vi "main(Test DQMH modules).vi"() -> ()   [LabVIEW 2018, in "Application.lvlib"] (continued)
              n2421 = call "App enquece.vi"("Priority Enquece"=TRUE, "command data"=w5478, "command"=w5479, "queue in"=w5481) -> ("error out"=w5482:errorcluster)  [unwired: 6 in, 1 out]
            }
          }
          frame True {
          }
        }
        n2422 = Merge Errors(w5454, w5456) -> (w5455:errorcluster)
      }
      frame "Test DRV 47" {
        w5488 = 47  # DUT index(0-59)
        n2423 = disable-structure shown="LOGGING==TRUE" {
          disable-tunnel: w5490 -> [w5525 _]
          frame condition #0 (active) {
            n2424 = Empty String/Path?(string/path=w5525) -> (empty?=w5528:bool)
            n2425 = Select(t="Quece timeout", s=w5528, f=w5525) -> (s? t:f=w5524:string)
            n2426 = call "string log (SubVI).vi"("Enum"=enum16{"Init", "Log", "Read"}."Log", "state Name"=w5524) -> ()  [unwired: 8 in, 2 out]
          }
          frame condition #1 {
          }
        }
        n2427 = call "progress string(SubVI).vi"("String 3"=w5490, "String in"=w5491) -> ("String out"=w5492:string)  [unwired: 9 in]
        n2428 = call "FGV Driver Data.vi"("DUT index(1-60)"=w5488) -> ("DUT SC"=w5489:bool)  [unwired: 7 in, 3 out]
        n2429 = case shown="False" w5489 {
          tunnel: [w5517 _] -> w5497
          tunnel: w5494 -> [w5516 _]
          frame False {
            w5504 = T11 {"command"="", "command data"=variant} ("element")
            w5503 = "MEAS.mux6_1"
            n2430 = To Variant(anything=T4."mux6-1_channel0" ("mux6_1(3wires)_encode")) -> (Variant=w5502:variant)
            n2431 = To Variant(anything=T4."mux6_1_channel5_3" ("mux6_1(3wires)_encode")) -> (Variant=w5514:variant)
            n2432 = To Variant(anything=T4."mux6_1_channel5_2" ("mux6_1(3wires)_encode")) -> (Variant=w5512:variant)
            n2433 = Bundle By Name(cluster=w5504, "command"=w5503, "command data"=w5512) -> (w5511:T11)
            n2434 = Bundle By Name(cluster=w5504, "command"=w5503, "command data"=w5514) -> (w5510:T11)
            n2435 = Bundle By Name(cluster=w5504, "command"=w5503, "command data"=w5502) -> ()  [unwired: 1 out]
            n2436 = Bundle By Name(cluster=w5504, "command"="MEAS.DMM dual read") -> (w5508:T11)
            n2437 = Build Array(w5511, w5510, w5508) -> (w5506:T11[])
            n2438 = Reverse 1D Array(array=w5506) -> (reversed array=w5507:T11[])
            n2439 = for {
              tunnel: [w5523] -> w5517 mode=indexing
              tunnel: w5516 -> [w5522]
              tunnel: w5507 -> [w5521] mode=indexing
              n2440 = Unbundle By Name(w5521) -> ("command"=w5520:string, "command data"=w5519:variant)
              n2441 = call "App enquece.vi"("Priority Enquece"=TRUE, "command data"=w5519, "command"=w5520, "queue in"=w5522) -> ("error out"=w5523:errorcluster)  [unwired: 6 in, 1 out]
            }
          }
          frame True {
          }
        }
        n2442 = Merge Errors(w5495, w5497) -> (w5496:errorcluster)
      }
      frame "Test DRV 48" {
        w5530 = 48  # DUT index(0-59)
        n2443 = disable-structure shown="LOGGING==TRUE" {
          disable-tunnel: w5531 -> [w5566 _]
          frame condition #0 (active) {
            n2444 = Empty String/Path?(string/path=w5566) -> (empty?=w5569:bool)
            n2445 = Select(t="Quece timeout", s=w5569, f=w5566) -> (s? t:f=w5565:string)
            n2446 = call "string log (SubVI).vi"("Enum"=enum16{"Init", "Log", "Read"}."Log", "state Name"=w5565) -> ()  [unwired: 8 in, 2 out]
          }
          frame condition #1 {
          }
        }
        n2447 = call "progress string(SubVI).vi"("String 3"=w5531, "String in"=w5532) -> ("String out"=w5533:string)  [unwired: 9 in]
        n2448 = call "FGV Driver Data.vi"("DUT index(1-60)"=w5530) -> ("DUT SC"=w5529:bool)  [unwired: 7 in, 3 out]
        n2449 = case shown="False" w5529 {
          tunnel: [w5558 _] -> w5538
          tunnel: w5535 -> [w5557 _]
          frame False {
            w5545 = T11 {"command"="", "command data"=variant} ("element")
            w5544 = "MEAS.mux6_1"
            n2450 = To Variant(anything=T4."mux6-1_channel0" ("mux6_1(3wires)_encode")) -> (Variant=w5543:variant)
            n2451 = To Variant(anything=T4."mux6_1_channel6_3" ("mux6_1(3wires)_encode")) -> (Variant=w5555:variant)
            n2452 = To Variant(anything=T4."mux6_1_channel6_2" ("mux6_1(3wires)_encode")) -> (Variant=w5553:variant)
            n2453 = Bundle By Name(cluster=w5545, "command"=w5544, "command data"=w5553) -> (w5552:T11)
            n2454 = Bundle By Name(cluster=w5545, "command"=w5544, "command data"=w5555) -> (w5551:T11)
            n2455 = Bundle By Name(cluster=w5545, "command"=w5544, "command data"=w5543) -> ()  [unwired: 1 out]
            n2456 = Bundle By Name(cluster=w5545, "command"="MEAS.DMM dual read") -> (w5549:T11)
            n2457 = Build Array(w5552, w5551, w5549) -> (w5547:T11[])
            n2458 = Reverse 1D Array(array=w5547) -> (reversed array=w5548:T11[])
            n2459 = for {
              tunnel: [w5564] -> w5558 mode=indexing
              tunnel: w5557 -> [w5563]
              tunnel: w5548 -> [w5562] mode=indexing
              n2460 = Unbundle By Name(w5562) -> ("command"=w5561:string, "command data"=w5560:variant)
              n2461 = call "App enquece.vi"("Priority Enquece"=TRUE, "command data"=w5560, "command"=w5561, "queue in"=w5563) -> ("error out"=w5564:errorcluster)  [unwired: 6 in, 1 out]
            }
          }
          frame True {
          }
        }
        n2462 = Merge Errors(w5536, w5538) -> (w5537:errorcluster)
      }
      frame "Test DRV 49" {
        w5570 = 49  # DUT index(0-59)
        n2463 = disable-structure shown="LOGGING==TRUE" {
          disable-tunnel: w5572 -> [w5607 _]
          frame condition #0 (active) {
            n2464 = Empty String/Path?(string/path=w5607) -> (empty?=w5610:bool)
            n2465 = Select(t="Quece timeout", s=w5610, f=w5607) -> (s? t:f=w5606:string)
            n2466 = call "string log (SubVI).vi"("Enum"=enum16{"Init", "Log", "Read"}."Log", "state Name"=w5606) -> ()  [unwired: 8 in, 2 out]
          }
          frame condition #1 {
          }
        }
        n2467 = call "progress string(SubVI).vi"("String 3"=w5572, "String in"=w5573) -> ("String out"=w5574:string)  [unwired: 9 in]
        n2468 = call "FGV Driver Data.vi"("DUT index(1-60)"=w5570) -> ("DUT SC"=w5571:bool)  [unwired: 7 in, 3 out]
        n2469 = case shown="False" w5571 {
          tunnel: [w5599 _] -> w5579
          tunnel: w5576 -> [w5598 _]
          frame False {
            w5586 = T11 {"command"="", "command data"=variant} ("element")
            w5585 = "MEAS.mux6_1"
            n2470 = To Variant(anything=T4."mux6-1_channel0" ("mux6_1(3wires)_encode")) -> (Variant=w5584:variant)
            n2471 = To Variant(anything=T4."mux6_1_channel1_3" ("mux6_1(3wires)_encode")) -> (Variant=w5596:variant)
            n2472 = To Variant(anything=T4."mux6-1_channel1_2" ("mux6_1(3wires)_encode")) -> (Variant=w5594:variant)
            n2473 = Bundle By Name(cluster=w5586, "command"=w5585, "command data"=w5594) -> (w5593:T11)
            n2474 = Bundle By Name(cluster=w5586, "command"=w5585, "command data"=w5596) -> (w5592:T11)
            n2475 = Bundle By Name(cluster=w5586, "command"=w5585, "command data"=w5584) -> ()  [unwired: 1 out]
            n2476 = Bundle By Name(cluster=w5586, "command"="MEAS.DMM dual read") -> (w5590:T11)
            n2477 = Build Array(w5593, w5592, w5590) -> (w5588:T11[])
            n2478 = Reverse 1D Array(array=w5588) -> (reversed array=w5589:T11[])
            n2479 = for {
              tunnel: [w5605] -> w5599 mode=indexing
              tunnel: w5598 -> [w5604]
              tunnel: w5589 -> [w5603] mode=indexing
              n2480 = Unbundle By Name(w5603) -> ("command"=w5602:string, "command data"=w5601:variant)
              n2481 = call "App enquece.vi"("Priority Enquece"=TRUE, "command data"=w5601, "command"=w5602, "queue in"=w5604) -> ("error out"=w5605:errorcluster)  [unwired: 6 in, 1 out]
            }
          }
          frame True {
          }
        }
        n2482 = Merge Errors(w5577, w5579) -> (w5578:errorcluster)
      }
      frame "Test DRV 50" {
        w5611 = 50  # DUT index(0-59)
        n2483 = disable-structure shown="LOGGING==TRUE" {
          disable-tunnel: w5613 -> [w5648 _]
          frame condition #0 (active) {
            n2484 = Empty String/Path?(string/path=w5648) -> (empty?=w5651:bool)
            n2485 = Select(t="Quece timeout", s=w5651, f=w5648) -> (s? t:f=w5647:string)
            n2486 = call "string log (SubVI).vi"("Enum"=enum16{"Init", "Log", "Read"}."Log", "state Name"=w5647) -> ()  [unwired: 8 in, 2 out]
          }
          frame condition #1 {
          }
        }
        n2487 = call "progress string(SubVI).vi"("String 3"=w5613, "String in"=w5614) -> ("String out"=w5615:string)  [unwired: 9 in]
        n2488 = call "FGV Driver Data.vi"("DUT index(1-60)"=w5611) -> ("DUT SC"=w5612:bool)  [unwired: 7 in, 3 out]
        n2489 = case shown="False" w5612 {
          tunnel: [w5640 _] -> w5620
          tunnel: w5617 -> [w5639 _]
          frame False {
            w5627 = T11 {"command"="", "command data"=variant} ("element")
            w5626 = "MEAS.mux6_1"
            n2490 = To Variant(anything=T4."mux6-1_channel0" ("mux6_1(3wires)_encode")) -> (Variant=w5625:variant)
            n2491 = To Variant(anything=T4."mux6_1_channel2_3" ("mux6_1(3wires)_encode")) -> (Variant=w5637:variant)
            n2492 = To Variant(anything=T4."mux6_1_channel2_2" ("mux6_1(3wires)_encode")) -> (Variant=w5635:variant)
            n2493 = Bundle By Name(cluster=w5627, "command"=w5626, "command data"=w5635) -> (w5634:T11)
            n2494 = Bundle By Name(cluster=w5627, "command"=w5626, "command data"=w5637) -> (w5633:T11)
            n2495 = Bundle By Name(cluster=w5627, "command"=w5626, "command data"=w5625) -> ()  [unwired: 1 out]
            n2496 = Bundle By Name(cluster=w5627, "command"="MEAS.DMM dual read") -> (w5631:T11)
            n2497 = Build Array(w5634, w5633, w5631) -> (w5629:T11[])
            n2498 = Reverse 1D Array(array=w5629) -> (reversed array=w5630:T11[])
            n2499 = for {
              tunnel: [w5646] -> w5640 mode=indexing
              tunnel: w5639 -> [w5645]
              tunnel: w5630 -> [w5644] mode=indexing
              n2500 = Unbundle By Name(w5644) -> ("command"=w5643:string, "command data"=w5642:variant)
              n2501 = call "App enquece.vi"("Priority Enquece"=TRUE, "command data"=w5642, "command"=w5643, "queue in"=w5645) -> ("error out"=w5646:errorcluster)  [unwired: 6 in, 1 out]
            }
          }
          frame True {
          }
        }
        n2502 = Merge Errors(w5618, w5620) -> (w5619:errorcluster)
      }
      frame "Test DRV 51" {
        w5653 = 51  # DUT index(0-59)
        n2503 = disable-structure shown="LOGGING==TRUE" {
          disable-tunnel: w5654 -> [w5689 _]
          frame condition #0 (active) {
            n2504 = Empty String/Path?(string/path=w5689) -> (empty?=w5692:bool)
            n2505 = Select(t="Quece timeout", s=w5692, f=w5689) -> (s? t:f=w5688:string)
            n2506 = call "string log (SubVI).vi"("Enum"=enum16{"Init", "Log", "Read"}."Log", "state Name"=w5688) -> ()  [unwired: 8 in, 2 out]
          }
          frame condition #1 {
          }
        }
        n2507 = call "progress string(SubVI).vi"("String 3"=w5654, "String in"=w5655) -> ("String out"=w5656:string)  [unwired: 9 in]
        n2508 = call "FGV Driver Data.vi"("DUT index(1-60)"=w5653) -> ("DUT SC"=w5652:bool)  [unwired: 7 in, 3 out]
        n2509 = case shown="False" w5652 {
          tunnel: [w5681 _] -> w5661
          tunnel: w5658 -> [w5680 _]
          frame False {
            w5668 = T11 {"command"="", "command data"=variant} ("element")
            w5667 = "MEAS.mux6_1"
            n2510 = To Variant(anything=T4."mux6-1_channel0" ("mux6_1(3wires)_encode")) -> (Variant=w5666:variant)
            n2511 = To Variant(anything=T4."mux6_1_channel3_3" ("mux6_1(3wires)_encode")) -> (Variant=w5678:variant)
            n2512 = To Variant(anything=T4."mux6_1_channel3_2" ("mux6_1(3wires)_encode")) -> (Variant=w5676:variant)
            n2513 = Bundle By Name(cluster=w5668, "command"=w5667, "command data"=w5676) -> (w5675:T11)
            n2514 = Bundle By Name(cluster=w5668, "command"=w5667, "command data"=w5678) -> (w5674:T11)
            n2515 = Bundle By Name(cluster=w5668, "command"=w5667, "command data"=w5666) -> ()  [unwired: 1 out]
            n2516 = Bundle By Name(cluster=w5668, "command"="MEAS.DMM dual read") -> (w5672:T11)
            n2517 = Build Array(w5675, w5674, w5672) -> (w5670:T11[])
            n2518 = Reverse 1D Array(array=w5670) -> (reversed array=w5671:T11[])
            n2519 = for {
              tunnel: [w5687] -> w5681 mode=indexing
              tunnel: w5680 -> [w5686]
              tunnel: w5671 -> [w5685] mode=indexing
              n2520 = Unbundle By Name(w5685) -> ("command"=w5684:string, "command data"=w5683:variant)
              n2521 = call "App enquece.vi"("Priority Enquece"=TRUE, "command data"=w5683, "command"=w5684, "queue in"=w5686) -> ("error out"=w5687:errorcluster)  [unwired: 6 in, 1 out]
            }
          }
          frame True {
          }
        }
        n2522 = Merge Errors(w5659, w5661) -> (w5660:errorcluster)
      }
      frame "Test DRV 52" {
        w5694 = 52  # DUT index(0-59)
        n2523 = disable-structure shown="LOGGING==TRUE" {
          disable-tunnel: w5695 -> [w5730 _]
          frame condition #0 (active) {
            n2524 = Empty String/Path?(string/path=w5730) -> (empty?=w5733:bool)
            n2525 = Select(t="Quece timeout", s=w5733, f=w5730) -> (s? t:f=w5729:string)
            n2526 = call "string log (SubVI).vi"("Enum"=enum16{"Init", "Log", "Read"}."Log", "state Name"=w5729) -> ()  [unwired: 8 in, 2 out]
          }
          frame condition #1 {
          }
        }
        n2527 = call "progress string(SubVI).vi"("String 3"=w5695, "String in"=w5696) -> ("String out"=w5697:string)  [unwired: 9 in]
        n2528 = call "FGV Driver Data.vi"("DUT index(1-60)"=w5694) -> ("DUT SC"=w5693:bool)  [unwired: 7 in, 3 out]
        n2529 = case shown="False" w5693 {
          tunnel: [w5722 _] -> w5702
          tunnel: w5699 -> [w5721 _]
          frame False {
            w5709 = T11 {"command"="", "command data"=variant} ("element")
            w5708 = "MEAS.mux6_1"
            n2530 = To Variant(anything=T4."mux6-1_channel0" ("mux6_1(3wires)_encode")) -> (Variant=w5707:variant)
            n2531 = To Variant(anything=T4."mux6_1_channel4_3" ("mux6_1(3wires)_encode")) -> (Variant=w5719:variant)
            n2532 = To Variant(anything=T4."mux6_1_channel4_2" ("mux6_1(3wires)_encode")) -> (Variant=w5717:variant)
            n2533 = Bundle By Name(cluster=w5709, "command"=w5708, "command data"=w5717) -> (w5716:T11)
            n2534 = Bundle By Name(cluster=w5709, "command"=w5708, "command data"=w5719) -> (w5715:T11)
            n2535 = Bundle By Name(cluster=w5709, "command"=w5708, "command data"=w5707) -> ()  [unwired: 1 out]
            n2536 = Bundle By Name(cluster=w5709, "command"="MEAS.DMM dual read") -> (w5713:T11)
            n2537 = Build Array(w5716, w5715, w5713) -> (w5711:T11[])
            n2538 = Reverse 1D Array(array=w5711) -> (reversed array=w5712:T11[])
            n2539 = for {
              tunnel: [w5728] -> w5722 mode=indexing
              tunnel: w5721 -> [w5727]
              tunnel: w5712 -> [w5726] mode=indexing
              n2540 = Unbundle By Name(w5726) -> ("command"=w5725:string, "command data"=w5724:variant)
              n2541 = call "App enquece.vi"("Priority Enquece"=TRUE, "command data"=w5724, "command"=w5725, "queue in"=w5727) -> ("error out"=w5728:errorcluster)  [unwired: 6 in, 1 out]
            }
          }
          frame True {
          }
        }
        n2542 = Merge Errors(w5700, w5702) -> (w5701:errorcluster)
      }
      frame "Test DRV 53" {
        w5734 = 53  # DUT index(0-59)
        n2543 = disable-structure shown="LOGGING==TRUE" {
          disable-tunnel: w5736 -> [w5771 _]
          frame condition #0 (active) {
            n2544 = Empty String/Path?(string/path=w5771) -> (empty?=w5774:bool)
            n2545 = Select(t="Quece timeout", s=w5774, f=w5771) -> (s? t:f=w5770:string)
            n2546 = call "string log (SubVI).vi"("Enum"=enum16{"Init", "Log", "Read"}."Log", "state Name"=w5770) -> ()  [unwired: 8 in, 2 out]
          }
          frame condition #1 {
          }
        }
        n2547 = call "progress string(SubVI).vi"("String 3"=w5736, "String in"=w5737) -> ("String out"=w5738:string)  [unwired: 9 in]
        n2548 = call "FGV Driver Data.vi"("DUT index(1-60)"=w5734) -> ("DUT SC"=w5735:bool)  [unwired: 7 in, 3 out]
        n2549 = case shown="False" w5735 {
          tunnel: [w5763 _] -> w5743
          tunnel: w5740 -> [w5762 _]
          frame False {
            w5748 = T11 {"command"="", "command data"=variant} ("element")
            w5750 = "MEAS.mux6_1"
            n2550 = To Variant(anything=T4."mux6-1_channel0" ("mux6_1(3wires)_encode")) -> (Variant=w5749:variant)
            n2551 = To Variant(anything=T4."mux6_1_channel5_3" ("mux6_1(3wires)_encode")) -> (Variant=w5760:variant)
            n2552 = To Variant(anything=T4."mux6_1_channel5_2" ("mux6_1(3wires)_encode")) -> (Variant=w5758:variant)
            n2553 = Bundle By Name(cluster=w5748, "command"=w5750, "command data"=w5758) -> (w5757:T11)
            n2554 = Bundle By Name(cluster=w5748, "command"=w5750, "command data"=w5760) -> (w5756:T11)
            n2555 = Bundle By Name(cluster=w5748, "command"=w5750, "command data"=w5749) -> ()  [unwired: 1 out]
            n2556 = Bundle By Name(cluster=w5748, "command"="MEAS.DMM dual read") -> (w5754:T11)
            n2557 = Build Array(w5757, w5756, w5754) -> (w5752:T11[])
            n2558 = Reverse 1D Array(array=w5752) -> (reversed array=w5753:T11[])
            n2559 = for {
              tunnel: [w5769] -> w5763 mode=indexing
              tunnel: w5762 -> [w5768]
              tunnel: w5753 -> [w5767] mode=indexing
              n2560 = Unbundle By Name(w5767) -> ("command"=w5766:string, "command data"=w5765:variant)
              n2561 = call "App enquece.vi"("Priority Enquece"=TRUE, "command data"=w5765, "command"=w5766, "queue in"=w5768) -> ("error out"=w5769:errorcluster)  [unwired: 6 in, 1 out]
            }
          }
          frame True {
          }
        }
        n2562 = Merge Errors(w5741, w5743) -> (w5742:errorcluster)
      }
      frame "Test DRV 54" {
        w5776 = 54  # DUT index(0-59)
        n2563 = disable-structure shown="LOGGING==TRUE" {
          disable-tunnel: w5777 -> [w5812 _]
          frame condition #0 (active) {
            n2564 = Empty String/Path?(string/path=w5812) -> (empty?=w5815:bool)
            n2565 = Select(t="Quece timeout", s=w5815, f=w5812) -> (s? t:f=w5811:string)
            n2566 = call "string log (SubVI).vi"("Enum"=enum16{"Init", "Log", "Read"}."Log", "state Name"=w5811) -> ()  [unwired: 8 in, 2 out]
          }
          frame condition #1 {
          }
        }
        n2567 = call "progress string(SubVI).vi"("String 3"=w5777, "String in"=w5778) -> ("String out"=w5779:string)  [unwired: 9 in]
        n2568 = call "FGV Driver Data.vi"("DUT index(1-60)"=w5776) -> ("DUT SC"=w5775:bool)  [unwired: 7 in, 3 out]
        n2569 = case shown="False" w5775 {
          tunnel: [w5804 _] -> w5784
          tunnel: w5781 -> [w5803 _]
          frame False {
            w5791 = T11 {"command"="", "command data"=variant} ("element")
            w5790 = "MEAS.mux6_1"
            n2570 = To Variant(anything=T4."mux6-1_channel0" ("mux6_1(3wires)_encode")) -> (Variant=w5789:variant)
            n2571 = To Variant(anything=T4."mux6_1_channel6_3" ("mux6_1(3wires)_encode")) -> (Variant=w5801:variant)
            n2572 = To Variant(anything=T4."mux6_1_channel6_2" ("mux6_1(3wires)_encode")) -> (Variant=w5799:variant)
            n2573 = Bundle By Name(cluster=w5791, "command"=w5790, "command data"=w5799) -> (w5798:T11)
            n2574 = Bundle By Name(cluster=w5791, "command"=w5790, "command data"=w5801) -> (w5797:T11)
            n2575 = Bundle By Name(cluster=w5791, "command"=w5790, "command data"=w5789) -> ()  [unwired: 1 out]
            n2576 = Bundle By Name(cluster=w5791, "command"="MEAS.DMM dual read") -> (w5795:T11)
            n2577 = Build Array(w5798, w5797, w5795) -> (w5793:T11[])
            n2578 = Reverse 1D Array(array=w5793) -> (reversed array=w5794:T11[])
            n2579 = for {
              tunnel: [w5810] -> w5804 mode=indexing
              tunnel: w5803 -> [w5809]
              tunnel: w5794 -> [w5808] mode=indexing
              n2580 = Unbundle By Name(w5808) -> ("command"=w5807:string, "command data"=w5806:variant)
              n2581 = call "App enquece.vi"("Priority Enquece"=TRUE, "command data"=w5806, "command"=w5807, "queue in"=w5809) -> ("error out"=w5810:errorcluster)  [unwired: 6 in, 1 out]
            }
          }
          frame True {
          }
        }
        n2582 = Merge Errors(w5782, w5784) -> (w5783:errorcluster)
      }
      frame "Test DRV 55" {
        w5817 = 55  # DUT index(0-59)
        n2583 = disable-structure shown="LOGGING==TRUE" {
          disable-tunnel: w5818 -> [w5853 _]
          frame condition #0 (active) {
            n2584 = Empty String/Path?(string/path=w5853) -> (empty?=w5856:bool)
            n2585 = Select(t="Quece timeout", s=w5856, f=w5853) -> (s? t:f=w5852:string)
            n2586 = call "string log (SubVI).vi"("Enum"=enum16{"Init", "Log", "Read"}."Log", "state Name"=w5852) -> ()  [unwired: 8 in, 2 out]
          }
          frame condition #1 {
          }
        }
        n2587 = call "progress string(SubVI).vi"("String 3"=w5818, "String in"=w5819) -> ("String out"=w5820:string)  [unwired: 9 in]
        n2588 = call "FGV Driver Data.vi"("DUT index(1-60)"=w5817) -> ("DUT SC"=w5816:bool)  [unwired: 7 in, 3 out]
        n2589 = case shown="False" w5816 {
          tunnel: [w5845 _] -> w5825
          tunnel: w5822 -> [w5844 _]
          frame False {
            w5832 = T11 {"command"="", "command data"=variant} ("element")
            w5831 = "MEAS.mux6_1"
            n2590 = To Variant(anything=T4."mux6-1_channel0" ("mux6_1(3wires)_encode")) -> (Variant=w5830:variant)
            n2591 = To Variant(anything=T4."mux6_1_channel1_3" ("mux6_1(3wires)_encode")) -> (Variant=w5842:variant)
            n2592 = To Variant(anything=T4."mux6-1_channel1_2" ("mux6_1(3wires)_encode")) -> (Variant=w5840:variant)
            n2593 = Bundle By Name(cluster=w5832, "command"=w5831, "command data"=w5840) -> (w5839:T11)
            n2594 = Bundle By Name(cluster=w5832, "command"=w5831, "command data"=w5842) -> (w5838:T11)
            n2595 = Bundle By Name(cluster=w5832, "command"=w5831, "command data"=w5830) -> ()  [unwired: 1 out]
            n2596 = Bundle By Name(cluster=w5832, "command"="MEAS.DMM dual read") -> (w5836:T11)
            n2597 = Build Array(w5839, w5838, w5836) -> (w5834:T11[])
            n2598 = Reverse 1D Array(array=w5834) -> (reversed array=w5835:T11[])
            n2599 = for {
              tunnel: [w5851] -> w5845 mode=indexing
              tunnel: w5844 -> [w5850]
              tunnel: w5835 -> [w5849] mode=indexing
              n2600 = Unbundle By Name(w5849) -> ("command"=w5848:string, "command data"=w5847:variant)
              n2601 = call "App enquece.vi"("Priority Enquece"=TRUE, "command data"=w5847, "command"=w5848, "queue in"=w5850) -> ("error out"=w5851:errorcluster)  [unwired: 6 in, 1 out]
            }
          }
          frame True {
          }
        }
        n2602 = Merge Errors(w5823, w5825) -> (w5824:errorcluster)
      }
      frame "Test DRV 56" {
        w5858 = 56  # DUT index(0-59)
        n2603 = disable-structure shown="LOGGING==TRUE" {
          disable-tunnel: w5859 -> [w5894 _]
          frame condition #0 (active) {
            n2604 = Empty String/Path?(string/path=w5894) -> (empty?=w5897:bool)
            n2605 = Select(t="Quece timeout", s=w5897, f=w5894) -> (s? t:f=w5893:string)
            n2606 = call "string log (SubVI).vi"("Enum"=enum16{"Init", "Log", "Read"}."Log", "state Name"=w5893) -> ()  [unwired: 8 in, 2 out]
          }
          frame condition #1 {
          }
        }
        n2607 = call "progress string(SubVI).vi"("String 3"=w5859, "String in"=w5860) -> ("String out"=w5861:string)  [unwired: 9 in]
        n2608 = call "FGV Driver Data.vi"("DUT index(1-60)"=w5858) -> ("DUT SC"=w5857:bool)  [unwired: 7 in, 3 out]
        n2609 = case shown="False" w5857 {
          tunnel: [w5886 _] -> w5866
          tunnel: w5863 -> [w5885 _]
          frame False {
            w5873 = T11 {"command"="", "command data"=variant} ("element")
            w5872 = "MEAS.mux6_1"
            n2610 = To Variant(anything=T4."mux6-1_channel0" ("mux6_1(3wires)_encode")) -> (Variant=w5871:variant)
            n2611 = To Variant(anything=T4."mux6_1_channel2_3" ("mux6_1(3wires)_encode")) -> (Variant=w5883:variant)
            n2612 = To Variant(anything=T4."mux6_1_channel2_2" ("mux6_1(3wires)_encode")) -> (Variant=w5881:variant)
            n2613 = Bundle By Name(cluster=w5873, "command"=w5872, "command data"=w5881) -> (w5880:T11)
            n2614 = Bundle By Name(cluster=w5873, "command"=w5872, "command data"=w5883) -> (w5879:T11)
            n2615 = Bundle By Name(cluster=w5873, "command"=w5872, "command data"=w5871) -> ()  [unwired: 1 out]
            n2616 = Bundle By Name(cluster=w5873, "command"="MEAS.DMM dual read") -> (w5877:T11)
            n2617 = Build Array(w5880, w5879, w5877) -> (w5875:T11[])
            n2618 = Reverse 1D Array(array=w5875) -> (reversed array=w5876:T11[])
            n2619 = for {
              tunnel: [w5892] -> w5886 mode=indexing
              tunnel: w5885 -> [w5891]
              tunnel: w5876 -> [w5890] mode=indexing
              n2620 = Unbundle By Name(w5890) -> ("command"=w5889:string, "command data"=w5888:variant)
              n2621 = call "App enquece.vi"("Priority Enquece"=TRUE, "command data"=w5888, "command"=w5889, "queue in"=w5891) -> ("error out"=w5892:errorcluster)  [unwired: 6 in, 1 out]
            }
          }
          frame True {
          }
        }
        n2622 = Merge Errors(w5864, w5866) -> (w5865:errorcluster)
      }
      frame "Test DRV 57" {
        w5899 = 57  # DUT index(0-59)
        n2623 = disable-structure shown="LOGGING==TRUE" {
          disable-tunnel: w5900 -> [w5935 _]
          frame condition #0 (active) {
            n2624 = Empty String/Path?(string/path=w5935) -> (empty?=w5938:bool)
            n2625 = Select(t="Quece timeout", s=w5938, f=w5935) -> (s? t:f=w5934:string)
            n2626 = call "string log (SubVI).vi"("Enum"=enum16{"Init", "Log", "Read"}."Log", "state Name"=w5934) -> ()  [unwired: 8 in, 2 out]
          }
          frame condition #1 {
          }
        }
        n2627 = call "progress string(SubVI).vi"("String 3"=w5900, "String in"=w5901) -> ("String out"=w5902:string)  [unwired: 9 in]
        n2628 = call "FGV Driver Data.vi"("DUT index(1-60)"=w5899) -> ("DUT SC"=w5898:bool)  [unwired: 7 in, 3 out]
        n2629 = case shown="False" w5898 {
          tunnel: [w5927 _] -> w5907
          tunnel: w5904 -> [w5926 _]
          frame False {
            w5914 = T11 {"command"="", "command data"=variant} ("element")
            w5913 = "MEAS.mux6_1"
            n2630 = To Variant(anything=T4."mux6-1_channel0" ("mux6_1(3wires)_encode")) -> (Variant=w5912:variant)
            n2631 = To Variant(anything=T4."mux6_1_channel3_3" ("mux6_1(3wires)_encode")) -> (Variant=w5924:variant)
            n2632 = To Variant(anything=T4."mux6_1_channel3_2" ("mux6_1(3wires)_encode")) -> (Variant=w5922:variant)
            n2633 = Bundle By Name(cluster=w5914, "command"=w5913, "command data"=w5922) -> (w5921:T11)
            n2634 = Bundle By Name(cluster=w5914, "command"=w5913, "command data"=w5924) -> (w5920:T11)
            n2635 = Bundle By Name(cluster=w5914, "command"=w5913, "command data"=w5912) -> ()  [unwired: 1 out]
            n2636 = Bundle By Name(cluster=w5914, "command"="MEAS.DMM dual read") -> (w5918:T11)
            n2637 = Build Array(w5921, w5920, w5918) -> (w5916:T11[])
            n2638 = Reverse 1D Array(array=w5916) -> (reversed array=w5917:T11[])
            n2639 = for {
              tunnel: [w5933] -> w5927 mode=indexing
              tunnel: w5926 -> [w5932]
              tunnel: w5917 -> [w5931] mode=indexing
              n2640 = Unbundle By Name(w5931) -> ("command"=w5930:string, "command data"=w5929:variant)
              n2641 = call "App enquece.vi"("Priority Enquece"=TRUE, "command data"=w5929, "command"=w5930, "queue in"=w5932) -> ("error out"=w5933:errorcluster)  [unwired: 6 in, 1 out]
            }
          }
          frame True {
          }
        }
        n2642 = Merge Errors(w5905, w5907) -> (w5906:errorcluster)
      }
      frame "Test DRV 58" {
        w5940 = 58  # DUT index(0-59)
        n2643 = disable-structure shown="LOGGING==TRUE" {
          disable-tunnel: w5941 -> [w5976 _]
          frame condition #0 (active) {
            n2644 = Empty String/Path?(string/path=w5976) -> (empty?=w5979:bool)
            n2645 = Select(t="Quece timeout", s=w5979, f=w5976) -> (s? t:f=w5975:string)
            n2646 = call "string log (SubVI).vi"("Enum"=enum16{"Init", "Log", "Read"}."Log", "state Name"=w5975) -> ()  [unwired: 8 in, 2 out]
          }
          frame condition #1 {
          }
        }
        n2647 = call "progress string(SubVI).vi"("String 3"=w5941, "String in"=w5942) -> ("String out"=w5943:string)  [unwired: 9 in]
        n2648 = call "FGV Driver Data.vi"("DUT index(1-60)"=w5940) -> ("DUT SC"=w5939:bool)  [unwired: 7 in, 3 out]
        n2649 = case shown="False" w5939 {
          tunnel: [w5968 _] -> w5948
          tunnel: w5945 -> [w5967 _]
          frame False {
            w5955 = T11 {"command"="", "command data"=variant} ("element")
            w5954 = "MEAS.mux6_1"
            n2650 = To Variant(anything=T4."mux6-1_channel0" ("mux6_1(3wires)_encode")) -> (Variant=w5953:variant)
            n2651 = To Variant(anything=T4."mux6_1_channel4_3" ("mux6_1(3wires)_encode")) -> (Variant=w5965:variant)
            n2652 = To Variant(anything=T4."mux6_1_channel4_2" ("mux6_1(3wires)_encode")) -> (Variant=w5963:variant)
            n2653 = Bundle By Name(cluster=w5955, "command"=w5954, "command data"=w5963) -> (w5962:T11)
            n2654 = Bundle By Name(cluster=w5955, "command"=w5954, "command data"=w5965) -> (w5961:T11)
            n2655 = Bundle By Name(cluster=w5955, "command"=w5954, "command data"=w5953) -> ()  [unwired: 1 out]
            n2656 = Bundle By Name(cluster=w5955, "command"="MEAS.DMM dual read") -> (w5959:T11)
            n2657 = Build Array(w5962, w5961, w5959) -> (w5957:T11[])
            n2658 = Reverse 1D Array(array=w5957) -> (reversed array=w5958:T11[])
            n2659 = for {
              tunnel: [w5974] -> w5968 mode=indexing
              tunnel: w5967 -> [w5973]
              tunnel: w5958 -> [w5972] mode=indexing
              n2660 = Unbundle By Name(w5972) -> ("command"=w5971:string, "command data"=w5970:variant)
              n2661 = call "App enquece.vi"("Priority Enquece"=TRUE, "command data"=w5970, "command"=w5971, "queue in"=w5973) -> ("error out"=w5974:errorcluster)  [unwired: 6 in, 1 out]
            }
          }
          frame True {
          }
        }
        n2662 = Merge Errors(w5946, w5948) -> (w5947:errorcluster)
      }
      frame "Test DRV 59" {
        w5981 = 59  # DUT index(0-59)
        n2663 = disable-structure shown="LOGGING==TRUE" {
          disable-tunnel: w5982 -> [w6017 _]
          frame condition #0 (active) {
            n2664 = Empty String/Path?(string/path=w6017) -> (empty?=w6020:bool)
            n2665 = Select(t="Quece timeout", s=w6020, f=w6017) -> (s? t:f=w6016:string)
            n2666 = call "string log (SubVI).vi"("Enum"=enum16{"Init", "Log", "Read"}."Log", "state Name"=w6016) -> ()  [unwired: 8 in, 2 out]
          }
          frame condition #1 {
          }
        }
        n2667 = call "progress string(SubVI).vi"("String 3"=w5982, "String in"=w5983) -> ("String out"=w5984:string)  [unwired: 9 in]
        n2668 = call "FGV Driver Data.vi"("DUT index(1-60)"=w5981) -> ("DUT SC"=w5980:bool)  [unwired: 7 in, 3 out]
        n2669 = case shown="False" w5980 {
          tunnel: [w6009 _] -> w5989
          tunnel: w5986 -> [w6008 _]
          frame False {
            w5996 = T11 {"command"="", "command data"=variant} ("element")
            w5995 = "MEAS.mux6_1"
            n2670 = To Variant(anything=T4."mux6-1_channel0" ("mux6_1(3wires)_encode")) -> (Variant=w5994:variant)
            n2671 = To Variant(anything=T4."mux6_1_channel5_3" ("mux6_1(3wires)_encode")) -> (Variant=w6006:variant)
            n2672 = To Variant(anything=T4."mux6_1_channel5_2" ("mux6_1(3wires)_encode")) -> (Variant=w6004:variant)
            n2673 = Bundle By Name(cluster=w5996, "command"=w5995, "command data"=w6004) -> (w6003:T11)
            n2674 = Bundle By Name(cluster=w5996, "command"=w5995, "command data"=w6006) -> (w6002:T11)
            n2675 = Bundle By Name(cluster=w5996, "command"=w5995, "command data"=w5994) -> ()  [unwired: 1 out]
            n2676 = Bundle By Name(cluster=w5996, "command"="MEAS.DMM dual read") -> (w6000:T11)
            n2677 = Build Array(w6003, w6002, w6000) -> (w5998:T11[])
            n2678 = Reverse 1D Array(array=w5998) -> (reversed array=w5999:T11[])
            n2679 = for {
              tunnel: [w6015] -> w6009 mode=indexing
              tunnel: w6008 -> [w6014]
              tunnel: w5999 -> [w6013] mode=indexing
              n2680 = Unbundle By Name(w6013) -> ("command"=w6012:string, "command data"=w6011:variant)
              n2681 = call "App enquece.vi"("Priority Enquece"=TRUE, "command data"=w6011, "command"=w6012, "queue in"=w6014) -> ("error out"=w6015:errorcluster)  [unwired: 6 in, 1 out]
            }
          }
          frame True {
          }
        }
        n2682 = Merge Errors(w5987, w5989) -> (w5988:errorcluster)
      }
      frame "Test DRV 60" {
        w6022 = 60  # DUT index(0-59)
        n2683 = disable-structure shown="LOGGING==TRUE" {
          disable-tunnel: w6023 -> [w6058 _]
          frame condition #0 (active) {
            n2684 = Empty String/Path?(string/path=w6058) -> (empty?=w6061:bool)
            n2685 = Select(t="Quece timeout", s=w6061, f=w6058) -> (s? t:f=w6057:string)
            n2686 = call "string log (SubVI).vi"("Enum"=enum16{"Init", "Log", "Read"}."Log", "state Name"=w6057) -> ()  [unwired: 8 in, 2 out]
          }
          frame condition #1 {
          }
        }
        n2687 = call "progress string(SubVI).vi"("String 3"=w6023, "String in"=w6024) -> ("String out"=w6025:string)  [unwired: 9 in]
        n2688 = call "FGV Driver Data.vi"("DUT index(1-60)"=w6022) -> ("DUT SC"=w6021:bool)  [unwired: 7 in, 3 out]
        n2689 = case shown="True" w6021 {
          tunnel: [w6050 _] -> w6030
          tunnel: w6027 -> [w6049 _]
          frame False {
            w6037 = T11 {"command"="", "command data"=variant} ("element")
            w6036 = "MEAS.mux6_1"
            n2690 = To Variant(anything=T4."mux6-1_channel0" ("mux6_1(3wires)_encode")) -> (Variant=w6035:variant)
            n2691 = To Variant(anything=T4."mux6_1_channel6_3" ("mux6_1(3wires)_encode")) -> (Variant=w6047:variant)
            n2692 = To Variant(anything=T4."mux6_1_channel6_2" ("mux6_1(3wires)_encode")) -> (Variant=w6045:variant)
            n2693 = Bundle By Name(cluster=w6037, "command"=w6036, "command data"=w6045) -> (w6044:T11)
            n2694 = Bundle By Name(cluster=w6037, "command"=w6036, "command data"=w6047) -> (w6043:T11)
            n2695 = Bundle By Name(cluster=w6037, "command"=w6036, "command data"=w6035) -> ()  [unwired: 1 out]
            n2696 = Bundle By Name(cluster=w6037, "command"="MEAS.DMM dual read") -> (w6041:T11)
            n2697 = Build Array(w6044, w6043, w6041) -> (w6039:T11[])
            n2698 = Reverse 1D Array(array=w6039) -> (reversed array=w6040:T11[])
            n2699 = for {
              tunnel: [w6056] -> w6050 mode=indexing
              tunnel: w6049 -> [w6055]
              tunnel: w6040 -> [w6054] mode=indexing
              n2700 = Unbundle By Name(w6054) -> ("command"=w6053:string, "command data"=w6052:variant)
              n2701 = call "App enquece.vi"("Priority Enquece"=TRUE, "command data"=w6052, "command"=w6053, "queue in"=w6055) -> ("error out"=w6056:errorcluster)  [unwired: 6 in, 1 out]
            }
          }
          frame True {
          }
        }
        n2702 = Merge Errors(w6028, w6030) -> (w6029:errorcluster)
      }
      frame "separated" {
      }
      frame "Test DRV 1A" {
        w6076 = T11 {"command"="", "command data"=variant} ("element")
        w6071 = 1 ("DUT index(0-59)")
        w6102 = T11 {"command"="", "command data"=variant} ("element")
        n2703 = disable-structure shown="LOGGING==TRUE" {
          disable-tunnel: w6080 -> [w6118 _]
          frame condition #0 (active) {
            n2704 = Empty String/Path?(string/path=w6118) -> (empty?=w6121:bool)
            n2705 = Select(t="Quece timeout", s=w6121, f=w6118) -> (s? t:f=w6117:string)
            n2706 = call "string log (SubVI).vi"("Enum"=enum16{"Init", "Log", "Read"}."Log", "state Name"=w6117) -> ()  [unwired: 8 in, 2 out]
          }
          frame condition #1 {
          }
        }
        n2707 = Flush Queue(queue=w6081) -> (queue out=w6082:refnum<queue>)  [unwired: 1 in, 2 out]
        n2708 = Decrement(x=w6071) -> (x-1=w6074:i32)
        n2709 = Index Array(array=w6070, index=w6074) -> (element=w6072:refnum<vi>)
        n2710 = property class="ColBox"(reference=w6072, "Value"=u32 10000536 ("DRV 1")) -> ()  [unwired: 1 in, 2 out]
        n2711 = To Variant(anything=bool[] [TRUE, FALSE, FALSE, FALSE, FALSE, FALSE]) -> (Variant=w6099:variant)
        n2712 = To Variant(anything=T6."demux1_10_channel1" ("demux1_10(x6)_encode")) -> (Variant=w6103:variant)
        n2713 = To Variant(anything=T4."mux6_1_channel1_3" ("mux6_1(3wires)_encode")) -> (Variant=w6107:variant)
        n2714 = To Variant(anything=T5."mux10_1_channel1" ("mux10_1(x6)_encode")) -> (Variant=w6109:variant)
        n2715 = Bundle By Name(cluster=w6102, "command"="MEAS.mux10-1", "command data"=w6109) -> (w6097:T11)
        n2716 = Bundle By Name(cluster=w6102, "command"="MEAS.mux6_1", "command data"=w6107) -> (w6096:T11)
        n2717 = Bundle By Name(cluster=w6102, "command"="MEAS.demux1-10", "command data"=w6103) -> (w6095:T11)
        n2718 = Bundle By Name(cluster=w6102, "command"="MEAS.eMIC", "command data"=w6099) -> (w6094:T11)
        n2719 = Bundle By Name(cluster=w6102, "command"="MEAS.AllRelaysOFF") -> (w6098:T11)
        n2720 = Build Array(w6098, w6097, w6096, w6095, w6094) -> (w6089:T11[])
        n2721 = Bundle By Name(cluster=w6076, "command"="MEAS.requestAC", "command data"=w6071) -> (w6090:T11)
        n2722 = Bundle By Name(cluster=w6076, "command"="Apps.WaitForEvent", "command data"=w6071) -> (w6075:T11)
        n2723 = Bundle By Name(cluster=w6076, "command"="MEAS.DMM dual read") -> (w6091:T11)
        n2724 = Bundle By Name(cluster=w6076, "command"="Apps.UI Update 1") -> (w6077:T11)
        n2725 = Build Array(w6091, w6090, w6075, w6077) -> (w6088:T11[])
        n2726 = Build Array (concatenate)(w6089, w6088) -> (w6087:T11[])
        n2727 = for {
          tunnel: w6087 -> [w6125] mode=indexing
          tunnel: w6082 -> [w6126]
          tunnel: [w6122] -> w6085 mode=indexing
          n2728 = Unbundle By Name(w6125) -> ("command"=w6124:string, "command data"=w6123:variant)
          n2729 = call "App enquece.vi"("command data"=w6123, "command"=w6124, "queue in"=w6126) -> ("error out"=w6122:errorcluster)  [unwired: 7 in, 1 out]
        }
        n2730 = Merge Errors(w6086, w6085) -> (w6084:errorcluster)
      }
      frame "Test DRV 2A" {
        w6133 = T11 {"command"="", "command data"=variant} ("element")
        w6128 = 2 ("DUT index(0-59)")
        w6159 = T11 {"command"="", "command data"=variant} ("element")
        n2731 = disable-structure shown="LOGGING==TRUE" {
          disable-tunnel: w6137 -> [w6175 _]
          frame condition #0 (active) {
            n2732 = Empty String/Path?(string/path=w6175) -> (empty?=w6178:bool)
            n2733 = Select(t="Quece timeout", s=w6178, f=w6175) -> (s? t:f=w6174:string)
            n2734 = call "string log (SubVI).vi"("Enum"=enum16{"Init", "Log", "Read"}."Log", "state Name"=w6174) -> ()  [unwired: 8 in, 2 out]
          }
          frame condition #1 {
          }
        }
        n2735 = Flush Queue(queue=w6138) -> (queue out=w6139:refnum<queue>)  [unwired: 1 in, 2 out]
        n2736 = Decrement(x=w6128) -> (x-1=w6131:i32)
        n2737 = Index Array(array=w6127, index=w6131) -> (element=w6129:refnum<vi>)
        n2738 = property class="ColBox"(reference=w6129, "Value"=u32 10000536 ("DRV 1")) -> ()  [unwired: 1 in, 2 out]
        n2739 = To Variant(anything=bool[] [FALSE, TRUE, FALSE, FALSE, FALSE, FALSE]) -> (Variant=w6156:variant)
        n2740 = To Variant(anything=T6."demux1_10_channel1" ("demux1_10(x6)_encode")) -> (Variant=w6160:variant)
        n2741 = To Variant(anything=T4."mux6_1_channel2_3" ("mux6_1(3wires)_encode")) -> (Variant=w6164:variant)
        n2742 = To Variant(anything=T5."mux10_1_channel1" ("mux10_1(x6)_encode")) -> (Variant=w6166:variant)
        n2743 = Bundle By Name(cluster=w6159, "command"="MEAS.mux10-1", "command data"=w6166) -> (w6154:T11)
        n2744 = Bundle By Name(cluster=w6159, "command"="MEAS.mux6_1", "command data"=w6164) -> (w6153:T11)
        n2745 = Bundle By Name(cluster=w6159, "command"="MEAS.demux1-10", "command data"=w6160) -> (w6152:T11)
        n2746 = Bundle By Name(cluster=w6159, "command"="MEAS.eMIC", "command data"=w6156) -> (w6151:T11)
        n2747 = Bundle By Name(cluster=w6159, "command"="MEAS.AllRelaysOFF") -> (w6155:T11)
        n2748 = Build Array(w6155, w6154, w6153, w6152, w6151) -> (w6146:T11[])
        n2749 = Bundle By Name(cluster=w6133, "command"="MEAS.requestAC", "command data"=w6128) -> (w6147:T11)
        n2750 = Bundle By Name(cluster=w6133, "command"="Apps.WaitForEvent", "command data"=w6128) -> (w6132:T11)
        n2751 = Bundle By Name(cluster=w6133, "command"="MEAS.DMM dual read") -> (w6148:T11)
        n2752 = Bundle By Name(cluster=w6133, "command"="Apps.UI Update 1") -> (w6134:T11)
        n2753 = Build Array(w6148, w6147, w6132, w6134) -> (w6145:T11[])
        n2754 = Build Array (concatenate)(w6146, w6145) -> (w6144:T11[])
        n2755 = for {
          tunnel: w6144 -> [w6182] mode=indexing
          tunnel: w6139 -> [w6183]
          tunnel: [w6179] -> w6142 mode=indexing
          n2756 = Unbundle By Name(w6182) -> ("command"=w6181:string, "command data"=w6180:variant)
          n2757 = call "App enquece.vi"("command data"=w6180, "command"=w6181, "queue in"=w6183) -> ("error out"=w6179:errorcluster)  [unwired: 7 in, 1 out]
        }
        n2758 = Merge Errors(w6143, w6142) -> (w6141:errorcluster)
      }
      frame "Test DRV 3A" {
        w6190 = T11 {"command"="", "command data"=variant} ("element")
        w6185 = 3 ("DUT index(0-59)")
        w6216 = T11 {"command"="", "command data"=variant} ("element")
        n2759 = disable-structure shown="LOGGING==TRUE" {
          disable-tunnel: w6194 -> [w6232 _]
          frame condition #0 (active) {
            n2760 = Empty String/Path?(string/path=w6232) -> (empty?=w6235:bool)
            n2761 = Select(t="Quece timeout", s=w6235, f=w6232) -> (s? t:f=w6231:string)
            n2762 = call "string log (SubVI).vi"("Enum"=enum16{"Init", "Log", "Read"}."Log", "state Name"=w6231) -> ()  [unwired: 8 in, 2 out]
          }
          frame condition #1 {
          }
        }
        n2763 = Flush Queue(queue=w6195) -> (queue out=w6196:refnum<queue>)  [unwired: 1 in, 2 out]
        n2764 = Decrement(x=w6185) -> (x-1=w6188:i32)
        n2765 = Index Array(array=w6184, index=w6188) -> (element=w6186:refnum<vi>)
        n2766 = property class="ColBox"(reference=w6186, "Value"=u32 10000536 ("DRV 1")) -> ()  [unwired: 1 in, 2 out]
        n2767 = To Variant(anything=bool[] [FALSE, FALSE, TRUE, FALSE, FALSE, FALSE]) -> (Variant=w6213:variant)
        n2768 = To Variant(anything=T6."demux1_10_channel1" ("demux1_10(x6)_encode")) -> (Variant=w6217:variant)
        n2769 = To Variant(anything=T4."mux6_1_channel3_3" ("mux6_1(3wires)_encode")) -> (Variant=w6221:variant)
        n2770 = To Variant(anything=T5."mux10_1_channel1" ("mux10_1(x6)_encode")) -> (Variant=w6223:variant)
        n2771 = Bundle By Name(cluster=w6216, "command"="MEAS.mux10-1", "command data"=w6223) -> (w6211:T11)
        n2772 = Bundle By Name(cluster=w6216, "command"="MEAS.mux6_1", "command data"=w6221) -> (w6210:T11)
        n2773 = Bundle By Name(cluster=w6216, "command"="MEAS.demux1-10", "command data"=w6217) -> (w6209:T11)
        n2774 = Bundle By Name(cluster=w6216, "command"="MEAS.eMIC", "command data"=w6213) -> (w6208:T11)
        n2775 = Bundle By Name(cluster=w6216, "command"="MEAS.AllRelaysOFF") -> (w6212:T11)
        n2776 = Build Array(w6212, w6211, w6210, w6209, w6208) -> (w6203:T11[])
        n2777 = Bundle By Name(cluster=w6190, "command"="MEAS.requestAC", "command data"=w6185) -> (w6204:T11)
        n2778 = Bundle By Name(cluster=w6190, "command"="Apps.WaitForEvent", "command data"=w6185) -> (w6189:T11)
        n2779 = Bundle By Name(cluster=w6190, "command"="MEAS.DMM dual read") -> (w6205:T11)
        n2780 = Bundle By Name(cluster=w6190, "command"="Apps.UI Update 1") -> (w6191:T11)
        n2781 = Build Array(w6205, w6204, w6189, w6191) -> (w6202:T11[])
        n2782 = Build Array (concatenate)(w6203, w6202) -> (w6201:T11[])
        n2783 = for {
          tunnel: w6201 -> [w6239] mode=indexing
          tunnel: w6196 -> [w6240]
          tunnel: [w6236] -> w6199 mode=indexing
          n2784 = Unbundle By Name(w6239) -> ("command"=w6238:string, "command data"=w6237:variant)
          n2785 = call "App enquece.vi"("command data"=w6237, "command"=w6238, "queue in"=w6240) -> ("error out"=w6236:errorcluster)  [unwired: 7 in, 1 out]
        }
        n2786 = Merge Errors(w6200, w6199) -> (w6198:errorcluster)
      }
      frame "Test DRV 4A" {
        w6247 = T11 {"command"="", "command data"=variant} ("element")
        w6241 = 4 ("DUT index(0-59)")
        w6273 = T11 {"command"="", "command data"=variant} ("element")
        n2787 = disable-structure shown="LOGGING==TRUE" {
          disable-tunnel: w6251 -> [w6289 _]
          frame condition #0 (active) {
            n2788 = Empty String/Path?(string/path=w6289) -> (empty?=w6292:bool)
            n2789 = Select(t="Quece timeout", s=w6292, f=w6289) -> (s? t:f=w6288:string)
            n2790 = call "string log (SubVI).vi"("Enum"=enum16{"Init", "Log", "Read"}."Log", "state Name"=w6288) -> ()  [unwired: 8 in, 2 out]
          }
          frame condition #1 {
          }
        }
        n2791 = Flush Queue(queue=w6252) -> (queue out=w6253:refnum<queue>)  [unwired: 1 in, 2 out]
        n2792 = Decrement(x=w6241) -> (x-1=w6245:i32)
        n2793 = Index Array(array=w6242, index=w6245) -> (element=w6243:refnum<vi>)
        n2794 = property class="ColBox"(reference=w6243, "Value"=u32 10000536 ("DRV 1")) -> ()  [unwired: 1 in, 2 out]
        n2795 = To Variant(anything=bool[] [FALSE, FALSE, FALSE, TRUE, FALSE, FALSE]) -> (Variant=w6270:variant)
        n2796 = To Variant(anything=T6."demux1_10_channel1" ("demux1_10(x6)_encode")) -> (Variant=w6274:variant)
        n2797 = To Variant(anything=T4."mux6_1_channel4_3" ("mux6_1(3wires)_encode")) -> (Variant=w6278:variant)
        n2798 = To Variant(anything=T5."mux10_1_channel1" ("mux10_1(x6)_encode")) -> (Variant=w6280:variant)
        n2799 = Bundle By Name(cluster=w6273, "command"="MEAS.mux10-1", "command data"=w6280) -> (w6268:T11)
        n2800 = Bundle By Name(cluster=w6273, "command"="MEAS.mux6_1", "command data"=w6278) -> (w6267:T11)
        n2801 = Bundle By Name(cluster=w6273, "command"="MEAS.demux1-10", "command data"=w6274) -> (w6266:T11)
        n2802 = Bundle By Name(cluster=w6273, "command"="MEAS.eMIC", "command data"=w6270) -> (w6265:T11)
        n2803 = Bundle By Name(cluster=w6273, "command"="MEAS.AllRelaysOFF") -> (w6269:T11)
        n2804 = Build Array(w6269, w6268, w6267, w6266, w6265) -> (w6260:T11[])
        n2805 = Bundle By Name(cluster=w6247, "command"="MEAS.requestAC", "command data"=w6241) -> (w6261:T11)
        n2806 = Bundle By Name(cluster=w6247, "command"="Apps.WaitForEvent", "command data"=w6241) -> (w6246:T11)
        n2807 = Bundle By Name(cluster=w6247, "command"="MEAS.DMM dual read") -> (w6262:T11)
        n2808 = Bundle By Name(cluster=w6247, "command"="Apps.UI Update 1") -> (w6248:T11)
        n2809 = Build Array(w6262, w6261, w6246, w6248) -> (w6259:T11[])
        n2810 = Build Array (concatenate)(w6260, w6259) -> (w6258:T11[])
        n2811 = for {
          tunnel: w6258 -> [w6296] mode=indexing
          tunnel: w6253 -> [w6297]
          tunnel: [w6293] -> w6256 mode=indexing
          n2812 = Unbundle By Name(w6296) -> ("command"=w6295:string, "command data"=w6294:variant)
          n2813 = call "App enquece.vi"("command data"=w6294, "command"=w6295, "queue in"=w6297) -> ("error out"=w6293:errorcluster)  [unwired: 7 in, 1 out]
        }
        n2814 = Merge Errors(w6257, w6256) -> (w6255:errorcluster)
      }
      frame "Test DRV 5A" {
        w6304 = T11 {"command"="", "command data"=variant} ("element")
        w6299 = 5 ("DUT index(0-59)")
        w6330 = T11 {"command"="", "command data"=variant} ("element")
        n2815 = disable-structure shown="LOGGING==TRUE" {
          disable-tunnel: w6308 -> [w6346 _]
          frame condition #0 (active) {
            n2816 = Empty String/Path?(string/path=w6346) -> (empty?=w6349:bool)
            n2817 = Select(t="Quece timeout", s=w6349, f=w6346) -> (s? t:f=w6345:string)
            n2818 = call "string log (SubVI).vi"("Enum"=enum16{"Init", "Log", "Read"}."Log", "state Name"=w6345) -> ()  [unwired: 8 in, 2 out]
          }
          frame condition #1 {
          }
        }
        n2819 = Flush Queue(queue=w6309) -> (queue out=w6310:refnum<queue>)  [unwired: 1 in, 2 out]
        n2820 = Decrement(x=w6299) -> (x-1=w6302:i32)
        n2821 = Index Array(array=w6298, index=w6302) -> (element=w6300:refnum<vi>)
        n2822 = property class="ColBox"(reference=w6300, "Value"=u32 10000536 ("DRV 1")) -> ()  [unwired: 1 in, 2 out]
        n2823 = To Variant(anything=bool[] [FALSE, FALSE, FALSE, FALSE, TRUE, FALSE]) -> (Variant=w6327:variant)
        n2824 = To Variant(anything=T6."demux1_10_channel1" ("demux1_10(x6)_encode")) -> (Variant=w6331:variant)
        n2825 = To Variant(anything=T4."mux6_1_channel5_3" ("mux6_1(3wires)_encode")) -> (Variant=w6335:variant)
        n2826 = To Variant(anything=T5."mux10_1_channel1" ("mux10_1(x6)_encode")) -> (Variant=w6337:variant)
        n2827 = Bundle By Name(cluster=w6330, "command"="MEAS.mux10-1", "command data"=w6337) -> (w6325:T11)
        n2828 = Bundle By Name(cluster=w6330, "command"="MEAS.mux6_1", "command data"=w6335) -> (w6324:T11)
        n2829 = Bundle By Name(cluster=w6330, "command"="MEAS.demux1-10", "command data"=w6331) -> (w6323:T11)
        n2830 = Bundle By Name(cluster=w6330, "command"="MEAS.eMIC", "command data"=w6327) -> (w6322:T11)
        n2831 = Bundle By Name(cluster=w6330, "command"="MEAS.AllRelaysOFF") -> (w6326:T11)
        n2832 = Build Array(w6326, w6325, w6324, w6323, w6322) -> (w6317:T11[])
        n2833 = Bundle By Name(cluster=w6304, "command"="MEAS.requestAC", "command data"=w6299) -> (w6318:T11)
